vi "String_to_Pathname.vi"(1 "Input String":string) -> (0 "path":path)   [LabVIEW 2015]
uses:
  Globals/Constants_global.vi
  Globals/Preference_global.vi
panel:
  out "size(s)":i32
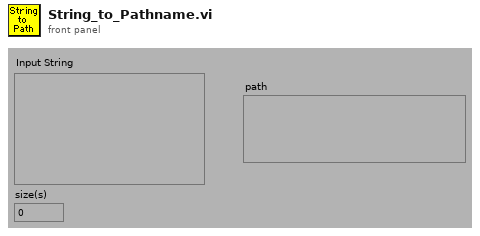
[diagram p1: front panel]
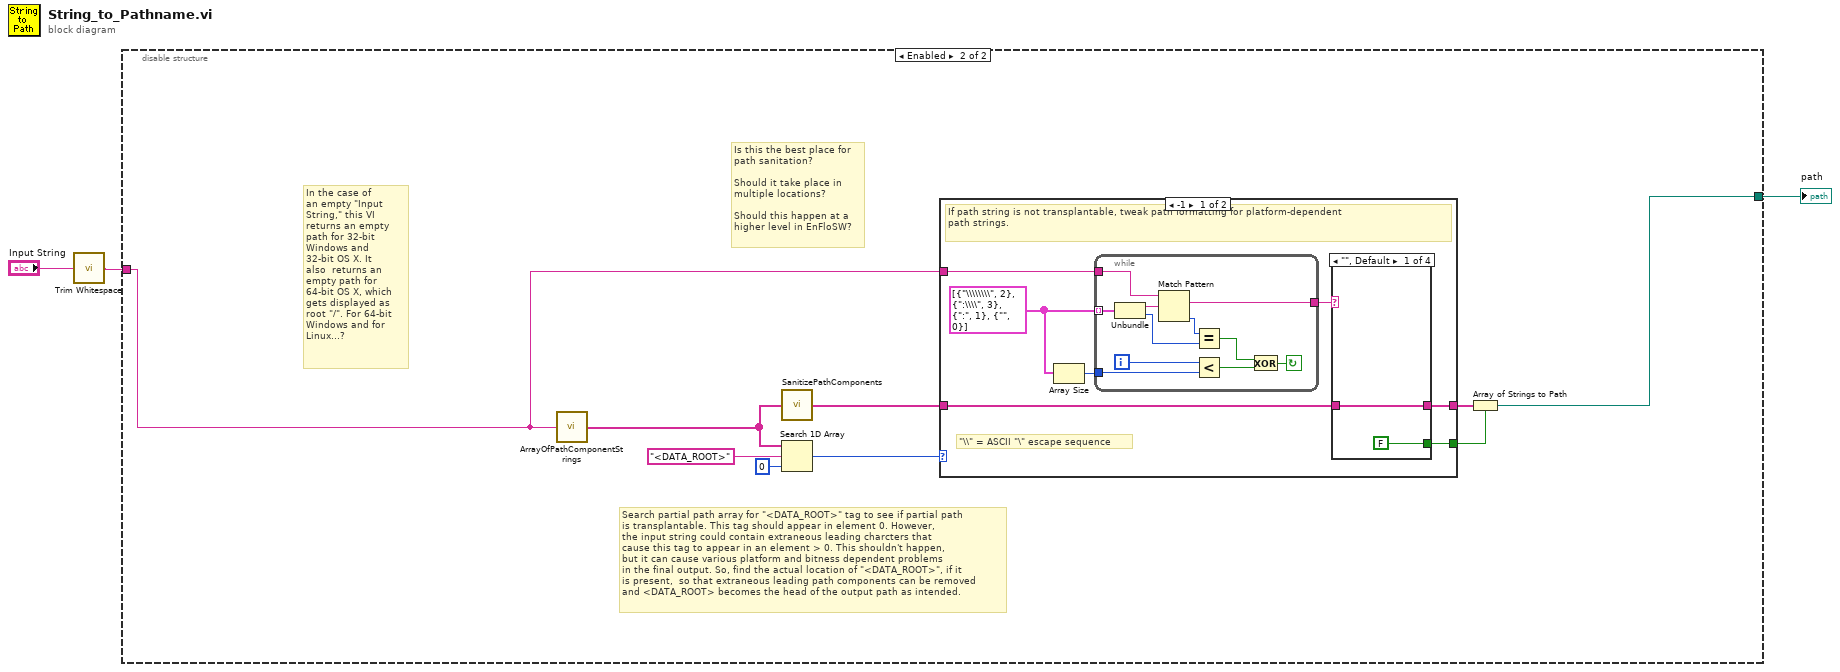
[diagram p0: block diagram]
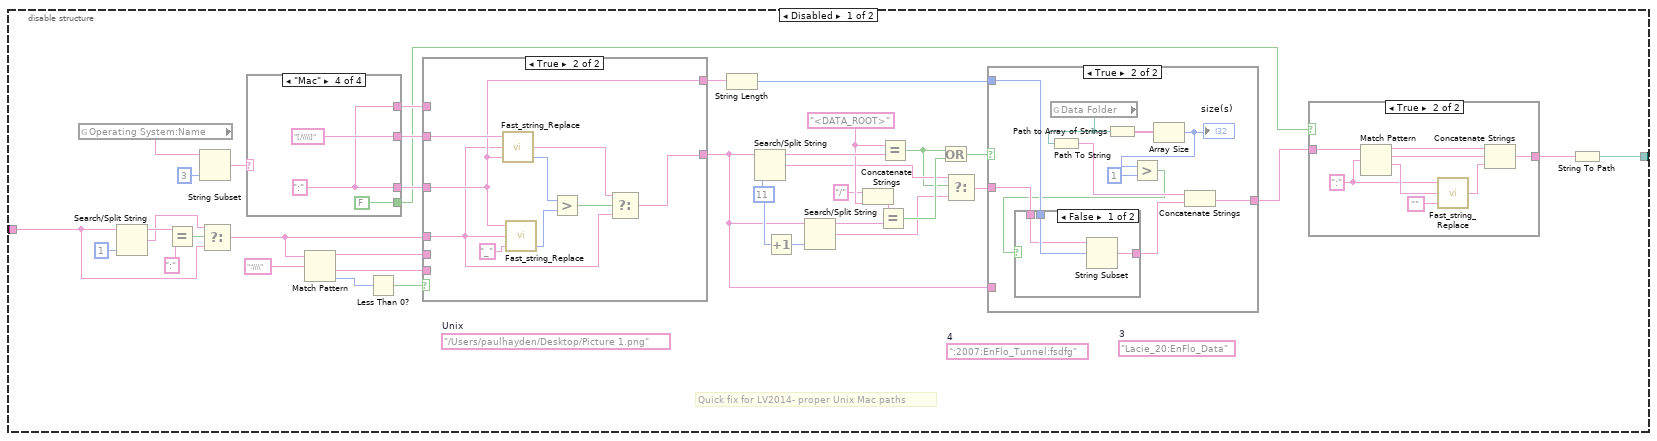
[diagram p2: hidden frame]
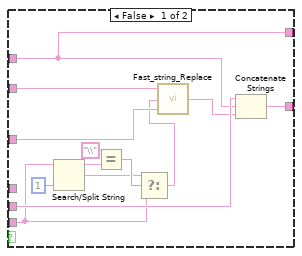
[diagram p6: hidden frame]
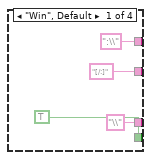
[diagram p7: hidden frame]
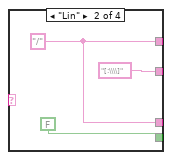
[diagram p8: hidden frame]
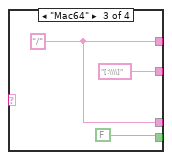
[diagram p9: hidden frame]
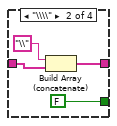
[diagram p10: hidden frame]
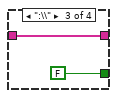
[diagram p11: hidden frame]
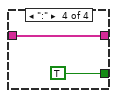
[diagram p12: hidden frame]
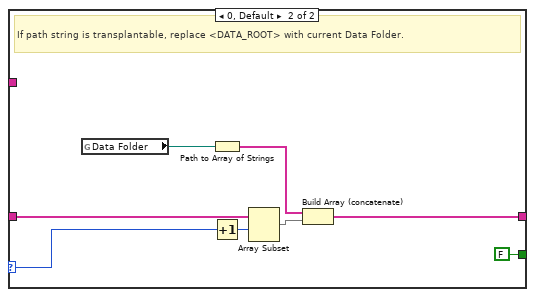
[diagram p13: hidden frame]
diagram:
  n1 = call <vilib>:"Trim Whitespace.vi"("string"="Input String") -> ("trimmed string"=w1:string)  [unwired: 1 in]
  n2 = disable-structure shown="Enabled" {
    disable-tunnel: [w24 w102] -> w3
    disable-tunnel: w1 -> [w4 w103]
    frame Disabled {
      (unwired) "Lacie_20:EnFlo_Data"  # 3
      (unwired) ":2007:EnFlo_Tunnel:fsdfg"  # 4
      (unwired) "/Users/paulhayden/Desktop/Picture 1.png"  # Unix
      w17 = 11
      w13 = "<DATA_ROOT>" ("regular expression")
      # "Quick fix for LV2014- proper Unix Mac paths"
      n3 = global read "Preference_global.vi" "Operating System:Name"() -> (w40:string)
      n4 = Search/Split String(string=w4, offset (0)=1 ("length (rest)")) -> (substring before match=w30:string, match + rest of string=w29:string)  [unwired: 2 out]
      n5 = Equal?(x=w30, y=":") -> (x = y?=w32:bool)
      n6 = String Subset(string=w40, length (rest)=3 ("length (rest)")) -> (substring=w41:string)  [unwired: 1 out]
      n7 = Select(t=w29, s=w32, f=w4) -> (s? t:f=w28:string)
      n8 = case shown="\"Mac\"" w41 {
        tunnel: ["[/:]" "[:\\\\]" "[:\\\\]" "[/\\\\]"] -> w35
        tunnel: ["\\" w93 w96 w99] -> w34
        tunnel: [":\\" w93 w96 w99] -> w23
        tunnel: [TRUE FALSE FALSE FALSE] -> w18
        frame "Win", Default {
        }
        frame "Lin" {
          w93 = "/"
        }
        frame "Mac64" {
          w96 = "/"
        }
        frame "Mac" {
          w99 = ":"
        }
      }
      n9 = Match Pattern(string=w28, regular expression=":\\\\") -> (before substring=w26:string, after substring=w27:string, offset past match=w37:i32)  [unwired: 2 out]
      n10 = Less Than 0?(x=w37) -> (x < 0?=w36:bool)
      n11 = case shown="True" w36 {
        tunnel: w28 -> [_ w80]
        tunnel: w35 -> [w78 w87]
        tunnel: w34 -> [w77 w86]
        tunnel: w27 -> [w67 _]
        tunnel: w26 -> [w76 _]
        tunnel: w23 -> [w73 _]
        tunnel: [w74 w79] -> w9
        tunnel: [w73 w86] -> w21
        frame False {
          n12 = Search/Split String(string=w67, offset (0)=1 ("length (rest)")) -> (substring before match=w71:string, match + rest of string=w68:string)  [unwired: 2 out]
          n13 = Equal?(x="\\", y=w71) -> (x = y?=w69:bool)
          n14 = Select(t=w68, s=w69, f=w67) -> (s? t:f=w66:string)
          n15 = call "Fast_string_Replace.vi"("Replace match with:"=w77, "Input String"=w66, "regular expression"=w78) -> ("Output String"=w75:string)  [unwired: 2 out]
          n16 = Concatenate Strings(w76, w73, w75) -> (w74:string)
        }
        frame True {
          n17 = call "Fast_string_Replace.vi"("Replace match with:"=w86, "Input String"=w80, "regular expression"=w87) -> ("Number Found"=w84:i32, "Output String"=w81:string)  [unwired: 1 out]
          n18 = call "Fast_string_Replace.vi"("Replace match with:"="_", "Input String"=w80, "regular expression"=w86) -> ("Number Found"=w83:i32)  [unwired: 2 out]
          n19 = Greater?(x=w84, y=w83) -> (0:w82:bool)
          n20 = Select(t=w81, s=w82, f=w80) -> (s? t:f=w79:string)
        }
      }
      n21 = String Length(string=w21) -> (length=w22:i32)
      n22 = Search/Split String(string=w9, offset (0)=w17) -> (substring before match=w25:string, match + rest of string=w6:string)  [unwired: 1 in, 1 out]
      n23 = Increment(x=w17) -> (x+1=w16:i32)
      n24 = Search/Split String(string=w9, offset (0)=w16) -> (substring before match=w15:string, match + rest of string=w7:string)  [unwired: 1 in, 1 out]
      n25 = Concatenate Strings("/" ("string"), w13) -> (w14:string)
      n26 = Equal?(x=w14, y=w15) -> (x = y?=w10:bool)
      n27 = Equal?(x=w13, y=w25) -> (x = y?=w5:bool)
      n28 = Or(x=w5, y=w10) -> (x .or. y?=w11:bool)
      n29 = Select(t=w6, s=w5, f=w7) -> (s? t:f=w8:string)
      n30 = case shown="True" w11 {
        tunnel: w9 -> [w51 _]
        tunnel: [w51 w55] -> w20
        tunnel: w8 -> [_ w59]
        tunnel: w22 -> [_ w60]
        frame False {
        }
        frame True {
          n31 = global read "Constants_global.vi" "Data Folder"() -> (w57:path)
          n32 = Path To String(path=w57) -> (string=w61:string)
          n33 = Path to Array of Strings(0:w57) -> (2:w56:string[])  [unwired: 1 out]
          n34 = Array Size(array=w56) -> (size(s)=w54:i32)
          "size(s)" <- w54
          n35 = Greater?(x=w54, y=1) -> (0:w52:bool)
          n36 = case shown="False" w52 {
            tunnel: w60 -> [w64 _]
            tunnel: w59 -> [w63 w65]
            tunnel: [w62 w65] -> w58
            frame False {
              n37 = String Subset(string=w63, offset (0)=w64) -> (substring=w62:string)  [unwired: 1 out]
            }
            frame True {
            }
          }
          n38 = Concatenate Strings(w61, w58) -> (w55:string)
        }
      }
      n39 = case shown="True" w18 {
        tunnel: w20 -> [w42 w50]
        tunnel: [w42 w43] -> w19
        frame False {
        }
        frame True {
          w48 = ":" ("regular expression")
          n40 = Match Pattern(string=w50, regular expression=w48) -> (before substring=w45:string, match substring=w44:string, after substring=w49:string)  [unwired: 2 out]
          n41 = call "Fast_string_Replace.vi"("Replace match with:"="", "Input String"=w49, "regular expression"=w48) -> ("Output String"=w46:string)  [unwired: 2 out]
          n42 = Concatenate Strings(w45, w44, w46) -> (w43:string)
        }
      }
      n43 = String To Path(string=w19) -> (path=w24:path)
    }
    frame Enabled {
      # "Is this the best place for\npath sanitation?\n\nShould it take place in\nmultiple locations?\n\nShould this happen at a\nhigher level in EnFloSW?"
      # "In the case of \nan empty \"Input \nString,\" this VI \nreturns an empty\npath for 32-bit\nWindows and\n32-bit OS X. It\nalso  returns an\nempty path for \n64-bit OS X, which\ngets displayed as\nroot \"/\". For 64-bit \nWindows and for\nLinux...?"
      # "Search partial path array for \"<DATA_ROOT>\" tag to see if partial path\nis transplantable. This tag should appear in element 0. However,\nthe input string could contain extraneous leading charcters that \ncause this tag to appear in an element > 0. This shouldn't happen,\nbut it can cause various platform and bitness dependent problems\nin the final output. So, find the actual location of \"<DATA_ROOT>\", if it\nis present,  so that extraneous leading path components can be removed\nand <DATA_ROOT> becomes the head of the output path as intended."
      n44 = call "ArrayOfPathComponentStrings.vi"("PathStringIn"=w103) -> ("ArrayOfPathComponentStringsOut"=w104:string[])
      n45 = call "SanitizePathComponents.vi"("PathComponentsIn"=w104) -> ("SanitizedComponentsOut"=w105:string[])
      n46 = Search 1D Array(1D array=w104, element="<DATA_ROOT>", start index (0)=0) -> (index of element=w101:i32)
      n47 = case shown="-1" w101 {
        selector: w101 -> [_ w141]
        tunnel: [w110 w145] -> w107
        tunnel: w105 -> [w111 w143]
        tunnel: [w112 FALSE] -> w106
        tunnel: w103 -> [w114 _]
        frame -1 {
          w115 = cluster{string, i32}[] [{"\\\\\\\\", 2}, {":\\\\", 3}, {":", 1}, {"", 0}]
          # "\"\\\\\" = ASCII \"\\\" escape sequence"
          # "If path string is not transplantable, tweak path formatting for platform-dependent\npath strings."
          n48 = Array Size(array=w115) -> (size(s)=w116:i32)
          n49 = while {
            tunnel: w115 -> [w129] mode=indexing
            tunnel: w116 -> [w137]
            tunnel: [w132] -> w113
            tunnel: w114 -> [w130]
            i -> [w131]
            stop <- w133 continue-if-true
            n50 = Unbundle(w129) -> (w127:string, w128:i32)
            n51 = Match Pattern(string=w130, regular expression=w127) -> (match substring=w132:string, offset past match=w135:i32)  [unwired: 1 in, 2 out]
            n52 = Equal?(x=w135, y=w128) -> (x = y?=w134:bool)
            n53 = Less?(x=w131, y=w137) -> (x < y?=w136:bool)
            n54 = Exclusive Or(1:w136, 2:w134) -> (0:w133:bool)
          }
          n55 = case shown="\"\", Default" w113 {
            tunnel: [FALSE FALSE FALSE TRUE] -> w112
            tunnel: w111 -> [w118 w119 w123 w125]
            tunnel: [w118 w120 w123 w125] -> w110
            frame "", Default {
            }
            frame "\\\\" {
              n56 = Build Array (concatenate)("\\", w119) -> (w120:string[])
            }
            frame ":\\" {
            }
            frame ":" {
            }
          }
        }
        frame 0, Default {
          # "If path string is transplantable, replace <DATA_ROOT> with current Data Folder."
          n57 = global read "Constants_global.vi" "Data Folder"() -> (w140:path)
          n58 = Path to Array of Strings(0:w140) -> (2:w139:string[])  [unwired: 1 out]
          n59 = Increment(x=w141) -> (x+1=w144:i32)
          n60 = Array Subset(array=w143, index=w144) -> (w142:string[])  [unwired: 1 in]
          n61 = Build Array (concatenate)(w139, w142) -> (w145:string[])
        }
      }
      n62 = Array of Strings to Path(0:w107, 1:w106) -> (2:w102:path)
    }
  }
  "path" <- w3
